vi "Final - PLC - Material Handling.vi"(9 "Timer preset (s)":dbl=6.0) -> (0 "Belt 1/2 \nin operation":bool, 6 "Current Timer (s)":dbl)   [LabVIEW 2014]
uses:
  <vilib>/Utility/file.llb/Write To Spreadsheet File (DBL).vi
panel:
  out "T1":bool
  out "M2-":bool
  out "M2+":bool
  out "M1-":bool
  out "M1+":bool
  out "?":bool
  out "D1":bool
  out "D0":bool
  out "D0":bool
  out "M2-":bool
  out "M2+":bool
  out "D1":bool
  out "D0":bool
  out "D0":bool
  out "M1-":bool
  out "M1+":bool
  out "T0":bool
  out "M0-":bool
  out "M0+":bool
  out "Start/Stop":bool
  out "D1":bool
  out "D1":bool
  out "T0":bool
  out "?":bool
  out "Start/Stop":bool
  in  "D0":bool
  in  "D1":bool
  in  "Start/Stop":bool
  out "M0-":bool
  out "M0+":bool
  out "W1":bool
  out "W2":bool
  out "W0":bool
  out "M1-":bool
  out "M1+":bool
  out "M2-":bool
  out "M2+":bool
  # "Ladder diagram"
  # "Sorter Control Panel"
  # "Timer T0"
  # "Belt 1"
  # "T0"
  # "#11"
  # "#10"
  # "Timer panel"
  # "Timer preset"
  # "Collection Zone 2"
  # "Collection Zone 1"
  # "Belt 0"
  # "BARCODE INPUT"
  # "Belt 2"
  # "#00"
  # "#01"
  # "Collection Zone 3"
  # "Collection Zone 4"
  # "Timer T1"
  # "T1"
  # "Timer preset"
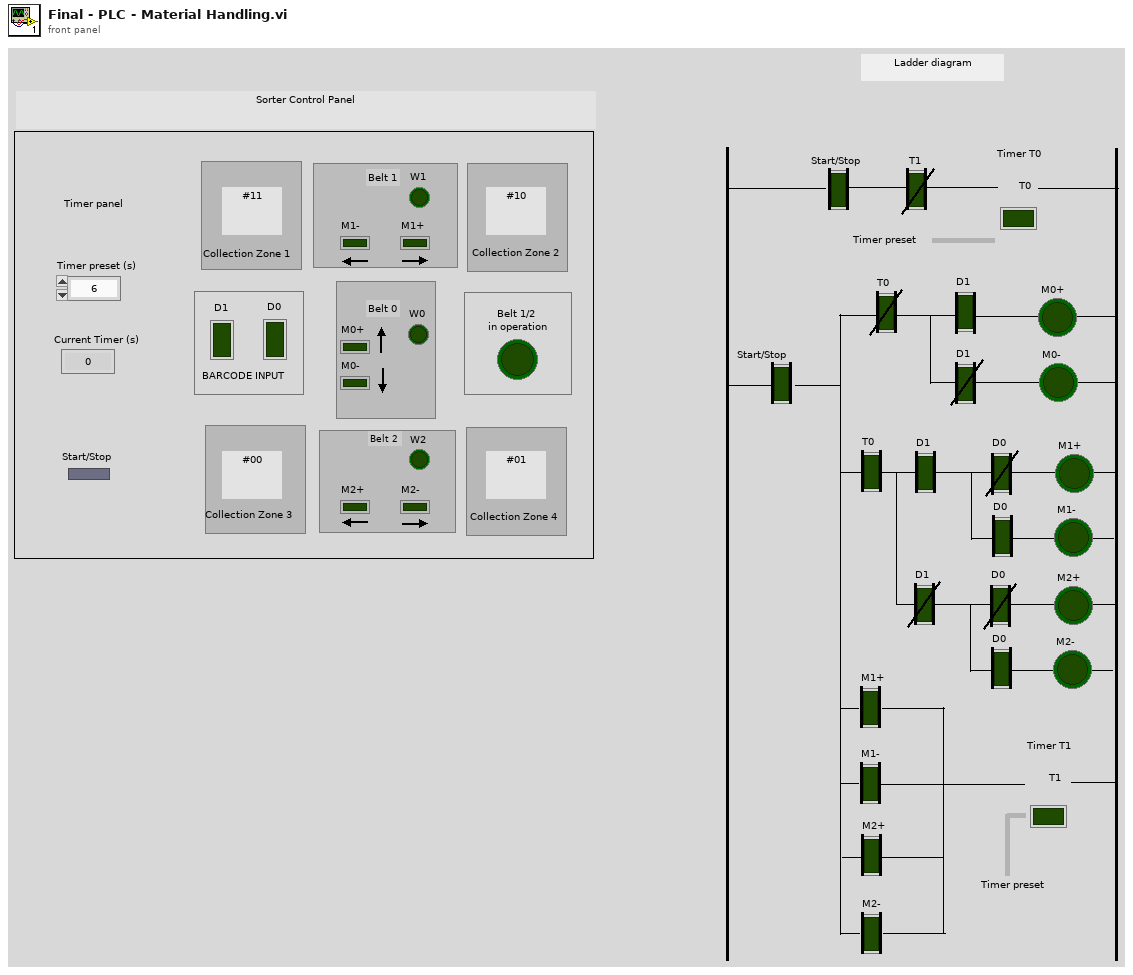
[diagram p1: front panel]
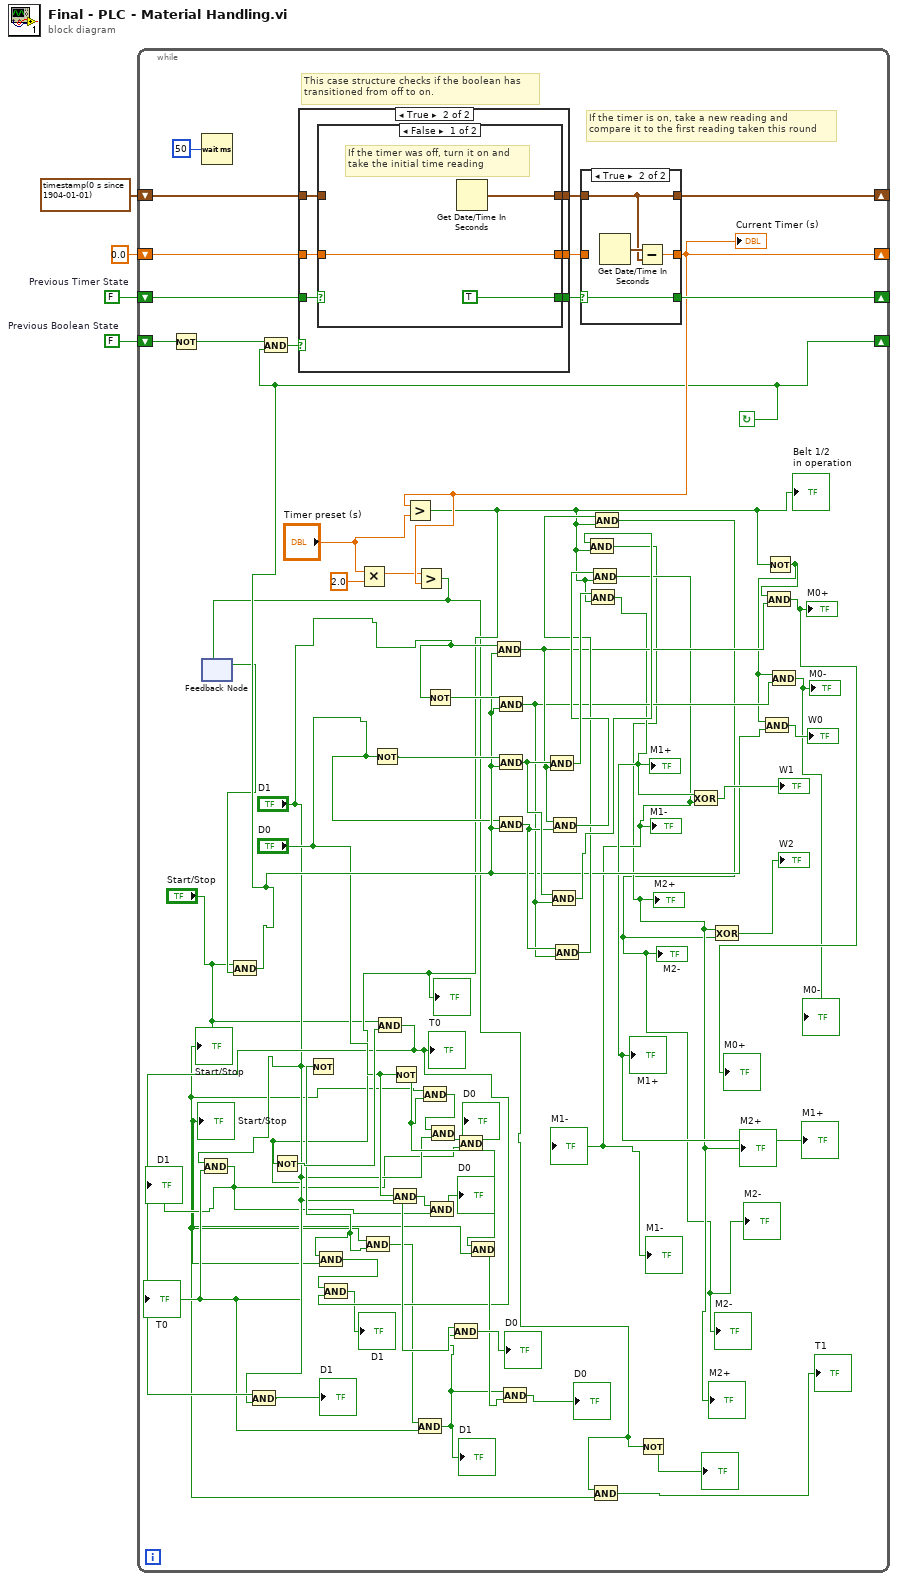
[diagram p0: block diagram]
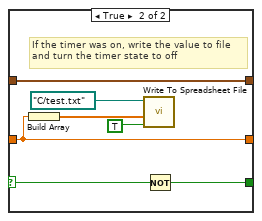
[diagram p4: hidden frame]
diagram:
  w2 = FALSE  # Previous Boolean State
  w4 = FALSE  # Previous Timer State
  n1 = while {
    shift-right: [w60] -> _
    shift-left: timestamp(0 s since 1904-01-01) ("seconds since 1Jan1904") -> [w59]
    shift-right: [w37] -> _
    shift-left: w2 -> [w66]
    shift-right: [w58] -> _
    shift-left: w4 -> [w63]
    shift-right: [w39] -> _
    shift-left: 0.0 -> [w57]
    stop <- w37 continue-if-true
    # "If the timer is on, take a new reading and \ncompare it to the first reading taken this round"
    # "This case structure checks if the boolean has\ntransitioned from off to on."
    n2 = Not(x=w66) -> (.not. x?=w65:bool)
    n3 = Wait (ms)(milliseconds to wait=u32 50) -> ()  [unwired: 1 out]
    n4 = feedback #1() -> (w36:bool)  [unwired: 1 in]
    n5 = And(x="Start/Stop", y=w36) -> (x .and. y?=w37:bool)
    n6 = And(x=w65, y=w37) -> (x .and. y?=w64:bool)
    n7 = case shown="True" w64 {
      tunnel: w63 -> [w77 w83]
      tunnel: [w76 w82] -> w62
      tunnel: [w77 w81] -> w61
      tunnel: w59 -> [w76 w80]
      tunnel: w57 -> [w75 w79]
      tunnel: [w75 w78] -> w56
      frame False {
      }
      frame True {
        n8 = case shown="False" w83 {
          selector: w83 -> [_ w91]
          tunnel: [w86 w93] -> w82
          tunnel: [TRUE w92] -> w81
          tunnel: w80 -> [_ w93]
          tunnel: w79 -> [w84 w90]
          tunnel: [w84 w90] -> w78
          frame False {
            # "If the timer was off, turn it on and \ntake the initial time reading"
            n9 = Get Date/Time In Seconds() -> (seconds since 1Jan1904=w86:timestamp)
          }
          frame True {
            # "If the timer was on, write the value to file\nand turn the timer state to off"
            n10 = Build Array(w90) -> (w89:dbl[])
            n11 = call-poly <vilib>:"Write To Spreadsheet File.vi"("append to file? (new file:F)"=TRUE, "1D data"=w89, "file path (dialog if empty)"=path "C:/test.txt") -> ()  [unwired: 5 in, 1 out]
            n12 = Not(x=w91) -> (.not. x?=w92:bool)
          }
        }
      }
    }
    n13 = Not(x="D1") -> (.not. x?=w28:bool)
    n14 = And(x=w28, y="Start/Stop") -> (x .and. y?=w20:bool)
    n15 = Multiply(x="Timer preset (s)", y=2.0) -> (x*y=w38:dbl)
    n16 = And(x="Start/Stop", y=w28) -> (x .and. y?=w17:bool)
    n17 = Not(x="D0") -> (.not. x?=w54:bool)
    n18 = And(x="D0", y="D1") -> (x .and. y?=w13:bool)
    n19 = Not(x="D0") -> (.not. x?=w27:bool)
    n20 = And(x="Start/Stop", y=w27) -> (x .and. y?=w26:bool)
    n21 = Not(x="D1") -> (.not. x?=w55:bool)
    n22 = And(x=w26, y="D1") -> (x .and. y?=w11:bool)
    n23 = And(x=w27, y="Start/Stop") -> (x .and. y?=w23:bool)
    n24 = And(x="D1", y=w37) -> (x .and. y?=w45:bool)
    n25 = And(x=w55, y=w37) -> (x .and. y?=w44:bool)
    n26 = And(x=w54, y=w37) -> (x .and. y?=w53:bool)
    n27 = And(x="D0", y=w37) -> (x .and. y?=w52:bool)
    n28 = And(x=w53, y=w45) -> (x .and. y?=w49:bool)
    n29 = And(x=w53, y=w44) -> (x .and. y?=w47:bool)
    n30 = And(x=w45, y=w52) -> (x .and. y?=w48:bool)
    n31 = And(x=w52, y=w44) -> (x .and. y?=w46:bool)
    n32 = case shown="True" w61 {
      selector: w61 -> [w69 w72]
      tunnel: w62 -> [w70 w73]
      tunnel: [w70 w73] -> w60
      tunnel: [w69 w72] -> w58
      tunnel: [w68 w71] -> w39
      tunnel: w56 -> [w68 _]
      frame False {
      }
      frame True {
        n33 = Get Date/Time In Seconds() -> (seconds since 1Jan1904=w74:timestamp)
        n34 = Subtract(x=w74, y=w73) -> (x-y=w71:dbl)
      }
    }
    "Current Timer (s)" <- w39
    n35 = Greater?(x=w39, y="Timer preset (s)") -> (0:w14:bool)
    "Belt 1/2 \nin operation" <- w14
    "?" <- w14
    "T0" <- w14
    n36 = And(x="D1", y=w14) -> (x .and. y?=w9:bool)
    "D1" <- w9
    n37 = Not(x=w14) -> (.not. x?=w29:bool)
    n38 = And(x="Start/Stop", y=w29) -> (x .and. y?=w19:bool)
    "T0" <- w19
    n39 = And(x=w19, y="D1") -> (x .and. y?=→"D1":bool)
    n40 = And(x=w20, y=w19) -> (x .and. y?=→"D1":bool)
    n41 = And(x=w17, y=w14) -> (x .and. y?=w16:bool)
    "D1" <- w16
    n42 = Greater?(x=w38, y=w39) -> (0:w7:bool)
    n43 = feedback-in #1(w7) -> ()
    n44 = And(x=w13, y=w9) -> (x .and. y?=→"D0":bool)
    n45 = And(x="D0", y=w16) -> (x .and. y?=→"D0":bool)
    n46 = And(x=w11, y=w9) -> (x .and. y?=→"D0":bool)
    n47 = And(x=w16, y=w23) -> (x .and. y?=→"D0":bool)
    n48 = And(x=w47, y=w14) -> (x .and. y?=w31:bool)
    "M2+" <- w31
    "M2+" <- w31
    "M2+" <- w31
    n49 = And(x=w49, y=w14) -> (x .and. y?=w33:bool)
    "M1+" <- w33
    "M1+" <- w33
    "M1+" <- w33
    n50 = And(x=w48, y=w14) -> (x .and. y?=w32:bool)
    "M1-" <- w32
    "M1-" <- w32
    "M1-" <- w32
    n51 = And(x=w7, y="Start/Stop") -> (x .and. y?=→"T1":bool)
    n52 = And(x=w46, y=w14) -> (x .and. y?=w30:bool)
    "M2-" <- w30
    "M2-" <- w30
    "M2-" <- w30
    n53 = Not(x=w7) -> (.not. x?=→"?":bool)
    n54 = Exclusive Or(1:w32, 2:w33) -> (0:→"W1":bool)
    n55 = Exclusive Or(1:w30, 2:w31) -> (0:→"W2":bool)
    n56 = Not(x=w14) -> (.not. x?=w43:bool)
    n57 = And(x=w43, y=w37) -> (x .and. y?=→"W0":bool)
    n58 = And(x=w43, y=w45) -> (x .and. y?=→"M0+" →"M0+":bool)
    n59 = And(x=w43, y=w44) -> (x .and. y?=→"M0-" →"M0-":bool)
    "Start/Stop" <- "Start/Stop"
    "Start/Stop" <- "Start/Stop"
  }
